vi "Global_Erros.vi"(6 "User Event In":refnum<user-event>, 7 "Action":T1, 9 "Error Loop 3":errorcluster, 10 "Error Loop2":errorcluster, 11 "Error Loop 1":errorcluster) -> (3 "User Event Out":refnum<user-event>)   [LabVIEW 2021, in "Main.lvlib"]
doc: "This Vi is used to collect the erros from the 4 loops and handle with them."
uses:
  Main.lvlib
  Tipski Definicii/error_handl.ctl
  subVIS/Main_Programs_SubVIs.lvlib
panel:
  # "Input"
  # "Output"
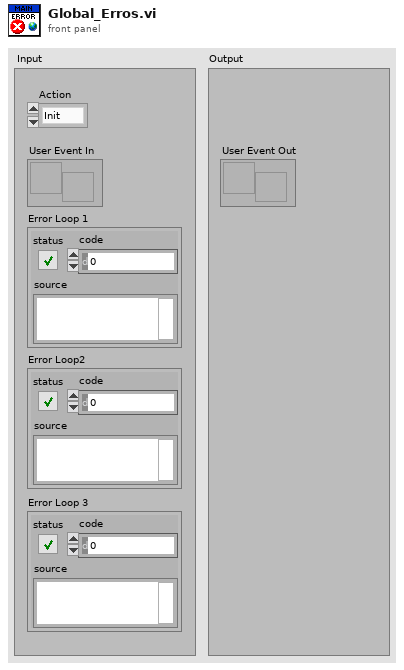
[diagram p1: front panel]
types:
  T1 = typedef "error_handl.ctl" = enum16{"Init", "Insert Error 1", "Insert Error 2", "Insert Error 3", "Insert Error 4", "Handle Erros"}
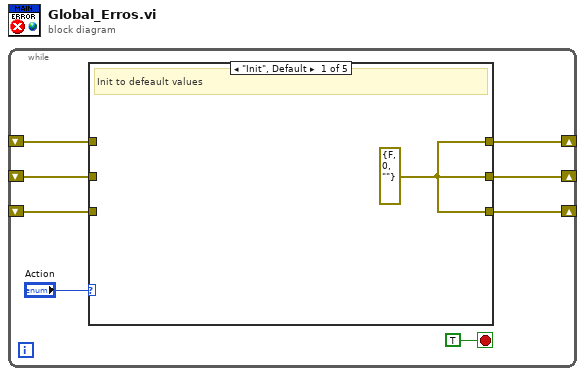
[diagram p0: block diagram]
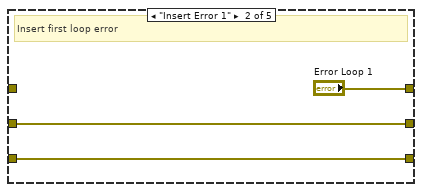
[diagram p2: hidden frame]
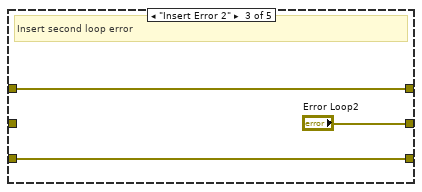
[diagram p3: hidden frame]
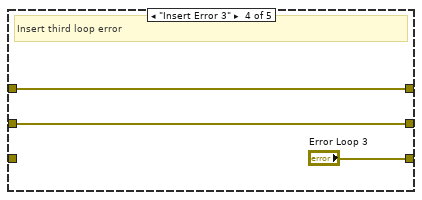
[diagram p4: hidden frame]
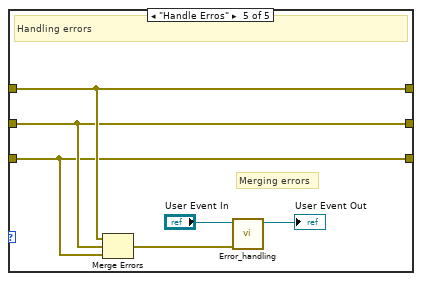
[diagram p5: hidden frame]
diagram:
  n1 = while {
    shift-right: [w6] -> _
    shift-left: _ -> [w5]
    shift-right: [w4] -> _
    shift-left: _ -> [w2]
    shift-right: [w3] -> _
    shift-left: _ -> [w1]
    stop <- TRUE stop-if-true
    n2 = case shown="\"Init\", Default" "Action" {
      tunnel: [w9 "Error Loop 1" w14 w18 w22] -> w6
      tunnel: w5 -> [_ _ w14 w18 w22]
      tunnel: [w9 w12 "Error Loop2" w17 w21] -> w4
      tunnel: [w9 w11 w13 "Error Loop 3" w20] -> w3
      tunnel: w2 -> [_ w12 _ w17 w21]
      tunnel: w1 -> [_ w11 w13 _ w20]
      frame "Init", Default {
        w9 = errorcluster {"status"=FALSE, "code"=0, "source"=""} ("error constant")
        # "Init to defeault values"
      }
      frame "Insert Error 1" {
        # "Insert first loop error"
      }
      frame "Insert Error 2" {
        # "Insert second loop error"
      }
      frame "Insert Error 3" {
        # "Insert third loop error"
      }
      frame "Handle Erros" {
        # "Merging errors"
        # "Handling errors"
        n3 = Merge Errors(w22, w21, w20) -> (w19:errorcluster)
        n4 = call "Error_handling.vi"("Error In"=w19, "User Event in"="User Event In") -> ("User Event out"=→"User Event Out":refnum<user-event>)  [unwired: 8 in, 1 out]
      }
    }
  }
